vi "DMA.Create Transfer (Single Block).vi"(8 "error in (no error)":errorcluster, 9 "RFM Offset":u32 format="%08x", 10 "Block Descriptor":T1 {"next descriptor ptr" format="%08x"; "data size" format="%08x"; "data ptr (upper)" format="%08x"; "data ptr (lower)" format="%08x"; "descriptor ptr (aligned)" format="%08x"; "descriptor size" format="%08x"; "descriptor ptr (VISA)" format="%08x"}, 11 "GE 5565PIORC in":refnum<class "GE 5565PIORC.lvclass">) -> (0 "error out":errorcluster, 1 "Transfer Size (bytes)":u32, 2 "DMA Transfer Spec":T2 {"Block Descriptors"."next descriptor ptr" format="%08x"; "Block Descriptors"."data size" format="%08x"; "Block Descriptors"."data ptr (upper)" format="%08x"; "Block Descriptors"."data ptr (lower)" format="%08x"; "Block Descriptors"."descriptor ptr (aligned)" format="%08x"; "Block Descriptors"."descriptor size" format="%08x"; "Block Descriptors"."descriptor ptr (VISA)" format="%08x"; "RFM Address" format="%08x"}, 3 "GE 5565PIORC out":refnum<class "GE 5565PIORC.lvclass">)   [LabVIEW 2016, in "GE 5565PIORC.lvclass"]
uses:
  GE 5565PIORC.lvclass
  Controls/DMA Transfer Spec.ctl
  Controls/DMA Block Descriptor.ctl
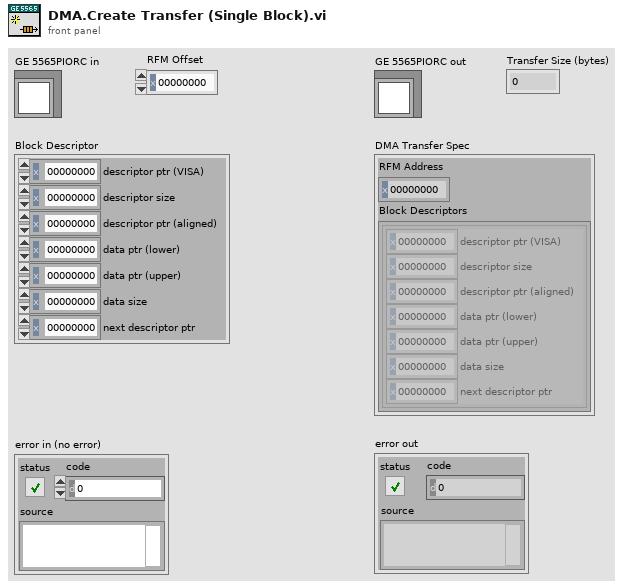
[diagram p1: front panel]
types:
  T1 = typedef "GE 5565PIORC.lvclass/DMA Block Descriptor.ctl" = cluster{"descriptor ptr (VISA)":u32, "descriptor size":u32, "descriptor ptr (aligned)":u32, "data ptr (lower)":u32, "data ptr (upper)":u32, "data size":u32, "next descriptor ptr":u32}
  T2 = typedef "GE 5565PIORC.lvclass/DMA Transfer Spec.ctl" = cluster{"RFM Address":u32, "Block Descriptors":T1[]}
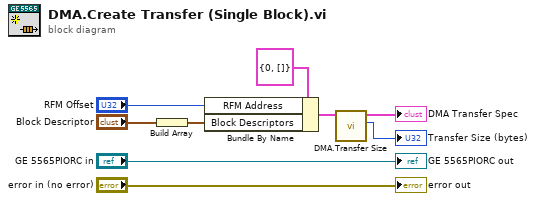
[diagram p0: block diagram]
diagram:
  n1 = Build Array("Block Descriptor") -> (w4:T1[])
  n2 = Bundle By Name(cluster=T2 {"RFM Address"=0, "Block Descriptors"=[]} ("DMA Transfer Spec"), "RFM Address"="RFM Offset", "Block Descriptors"=w4) -> (w3:T2)
  n3 = call "DMA.Transfer Size.vi"("DMA Transfer Spec"=w3) -> ("Transfer Size (bytes)"=→"Transfer Size (bytes)":u32, "DMA Transfer Spec out"=→"DMA Transfer Spec":T2)  [unwired: 9 in]
  "error out" <- "error in (no error)"
  "GE 5565PIORC out" <- "GE 5565PIORC in"
